vi "LV SCISDK Allocate Buffer Oscilloscope.vi"(7 "handle":u64, 8 "error in (no error)":errorcluster, 9 "buffer":T1, 10 "buffer_type":i32, 11 "Path":string) -> (0 "error out":errorcluster, 1 "buffer out":T1, 3 "function return":i32, 5 "handle out":u64)   [LabVIEW 2021, in "SciSDK_Labview.lvlib"]
doc: "SCISDKLABVIEW_DLL_API int LV_SCISDK_AllocateBuffer_Oscilloscope(char* Path, int buffer_type, LV_OSCILLOSCOPE_DECODED_BUFFER* buffer, void* handle);"
uses:
  SciSDK_Labview.lvlib
  <userlib>/SciSDK_Labview/SciSDK_Labview.dll
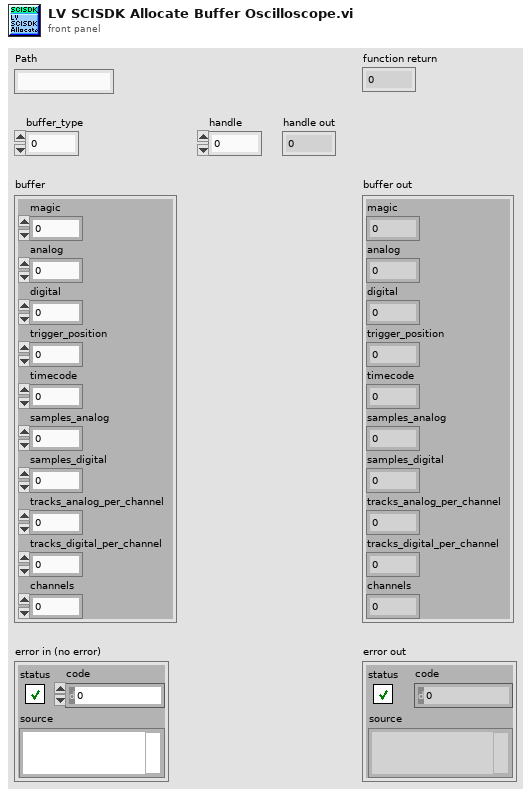
[diagram p1: front panel]
types:
  T1 = cluster{"magic":u32, "analog":u64, "digital":u64, "trigger_position":u32, "timecode":u32, "samples_analog":u32, "samples_digital":u32, "tracks_analog_per_channel":u32, "tracks_digital_per_channel":u32, "channels":u32}
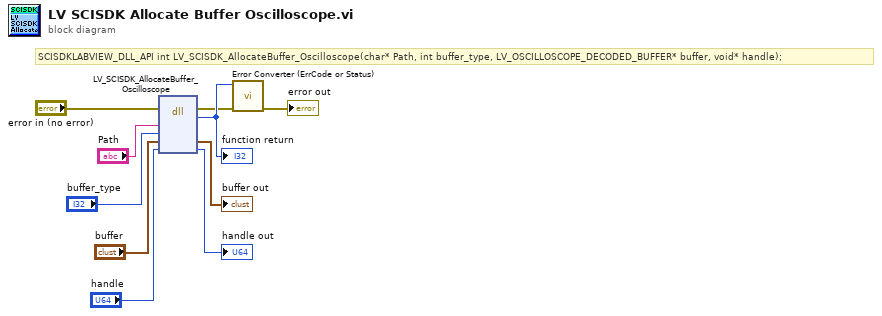
[diagram p0: block diagram]
diagram:
  # "SCISDKLABVIEW_DLL_API int LV_SCISDK_AllocateBuffer_Oscilloscope(char* Path, int buffer_type, LV_OSCILLOSCOPE_DECODED_BUFFER* buffer, void* handle);"
  n1 = dll-call lib="C:/Program Files/National Instruments/LabVIEW 2021/user.lib/SciSDK_Labview/SciSDK_Labview.*" fn="LV_SCISDK_AllocateBuffer_Oscilloscope"(error in="error in (no error)", "Path"="Path", "buffer_type"="buffer_type", "buffer"="buffer", "handle"="handle") -> (error out=w2:errorcluster, w10:i32, "buffer"=→"buffer out":T1, "handle"=→"handle out":u64)  [unwired: 4 in, 1 out]
  "function return" <- w10
  n2 = call <userlib>:"Error Converter (ErrCode or Status).vi"("error in (no error)"=w2, "error code"=w10) -> ("error out"=→"error out":errorcluster)  [unwired: 9 in]
